vi "CAN Set Relay.vi"(10 "RelayState":u8, 11 "DevHandle":i32) -> (3 "function return":i32)   [LabVIEW 2010, in "usb2can.lvlib"]
doc: "int WINAPI CAN_SetRelay(int DevHandle, unsigned char RelayState);"
uses:
  usb2can.lvlib
  USB2XXX.dll
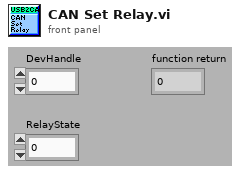
[diagram p1: front panel]
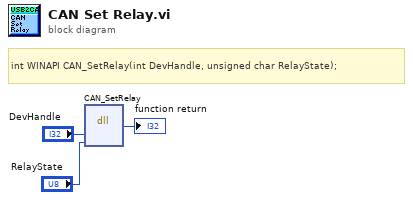
[diagram p0: block diagram]
diagram:
  # "int WINAPI CAN_SetRelay(int DevHandle, unsigned char RelayState);"
  n1 = dll-call lib="E:/Projects/USB2XXX_Example/sdk/api/Labview/usb2can/USB2XXX.*" fn="CAN_SetRelay"("DevHandle"="DevHandle", "RelayState"="RelayState") -> (→"function return":i32)  [unwired: 5 in, 2 out]
